vi "GetTagListing.vi"(8 "error in (no error)":errorcluster) -> (0 "error out":errorcluster, 2 "info":string[][](array[string]), 3 "tags":string[](array[string]))   [LabVIEW 2020]
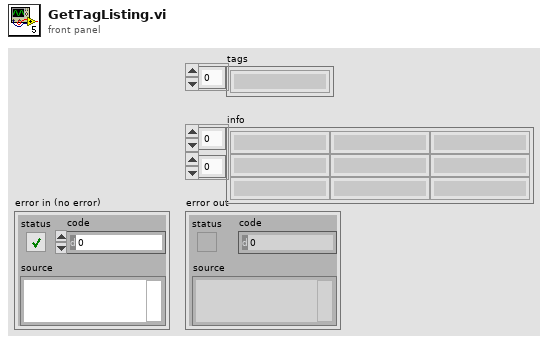
[diagram p1: front panel]
types:
  T1 = enum16{"GET", "PUT", "POST", "MultiPOST", "DELETE"}
  T2 = cluster{"tagsWithValues":cluster{"tag":cluster{"path":string, "type":string}, "current":cluster{"timestamp":string, "value":cluster{"type":string, "value":string}}}[]}
  T3 = cluster{"Name":string, "BaseURL":string, "AppKey":string, "Headers":string[], "Timeout":i32}
  T4 = cluster{"url":string, "sent headers":string, "sent body":string, "headers":string, "body":string, "Sent":string, "Received":string}
  T5 = cluster{"tag":cluster{"path":string, "type":string}, "current":cluster{"timestamp":string, "value":cluster{"type":string, "value":string}}}[]
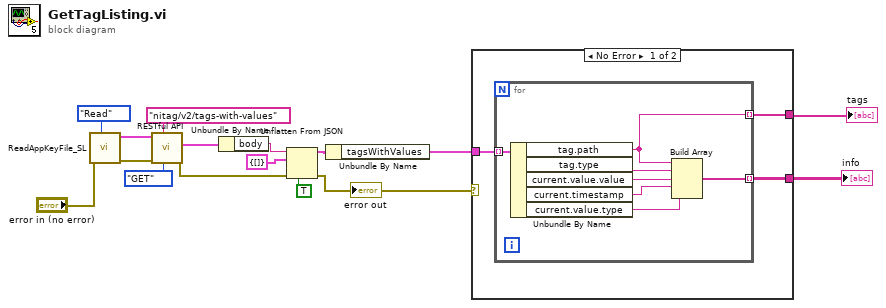
[diagram p0: block diagram]
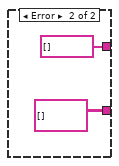
[diagram p2: hidden frame]
diagram:
  n1 = call "ReadAppKeyFile_SL.vi"("Task"=enum16{"Read", "Write"}."Read", "error in (no error)"="error in (no error)") -> ("error out"=w1:errorcluster, "Device Out"=w9:T3)  [unwired: 7 in, 1 out]
  n2 = call "RESTful API.vi"("Method"=T1."GET", "url"="nitag/v2/tags-with-values", "error in"=w1, "Device In"=w9) -> ("error out"=w12:errorcluster, "Comm"=w11:T4)  [unwired: 5 in, 1 out]
  n3 = Unbundle By Name(w11) -> ("body"=w6:string)
  n4 = Unflatten From JSON(JSON string=w6, type and defaults=T2 {"tagsWithValues"=[]}, default null elements? (F)=TRUE, error in (no error)=w12) -> (value=w3:T2, error out=w7:errorcluster)  [unwired: 3 in]
  "error out" <- w7
  n5 = Unbundle By Name(w3) -> ("tagsWithValues"=w5:T5)
  n6 = case shown="No Error" w7 {
    tunnel: w5 -> [w19 _]
    tunnel: [w18 string[][] []] -> w14
    tunnel: [w17 string[] []] -> w16
    frame No Error {
      n7 = for {
        tunnel: w19 -> [w26] mode=indexing
        tunnel: [w21] -> w18 mode=indexing
        tunnel: [w20] -> w17 mode=indexing
        n8 = Unbundle By Name(w26) -> ("tag.path"=w20:string, "tag.type"=w25:string, "current.value.value"=w24:string, "current.timestamp"=w23:string, "current.value.type"=w22:string)
        n9 = Build Array(w20, w25, w24, w23, w22) -> (w21:string[])
      }
    }
    frame Error {
    }
  }
  "tags" <- w16
  "info" <- w14
